vi "Setup_time_windows.vi"() -> ()   [LabVIEW 2017]
uses:
  <vilib>/Utility/file.llb/Read Delimited Spreadsheet (I64).vi
panel:
  in  "x":dbl=25000.0 format="%#_13g"
  out "x/y":dbl=0.25
  out "cal 2":dbl[][](graph)
  out "x-y":dbl
  in  "fine":u64=192 format="%x"
  out "time":dbl=25000.0 format="%.000f"
  in  "通道数量":i32=128
  in  "ch list":u16[](array[numeric])=[0, 1, 6, 7]
  in  "codeDensity":path=path "G:/tdc/2017/test_20240419_071836_codeDensity.csv"
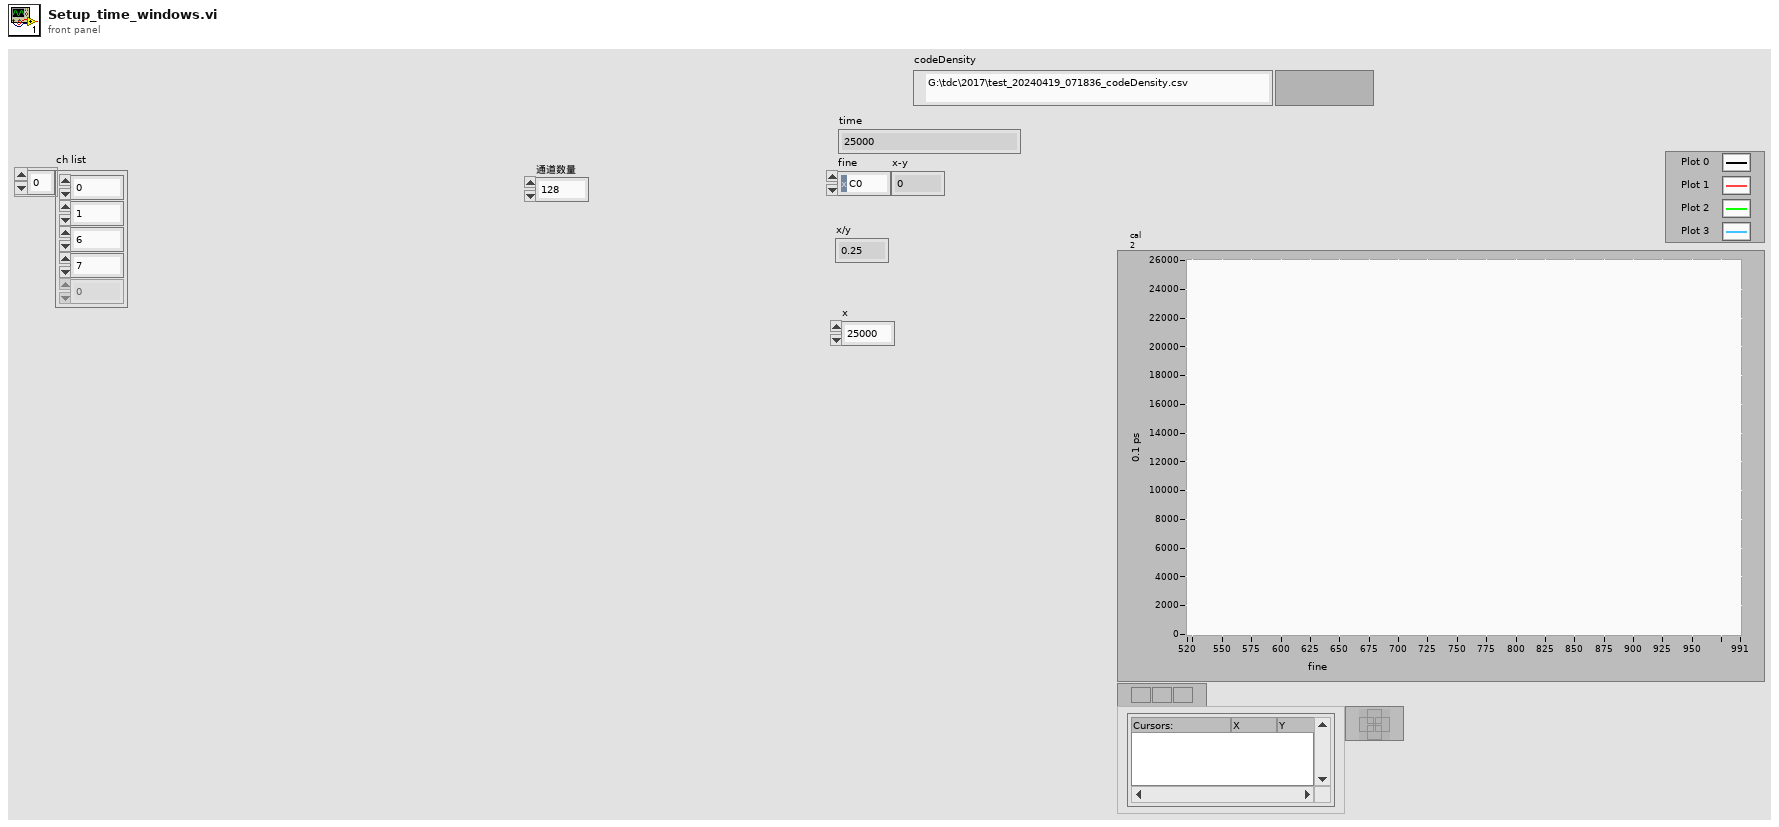
[diagram p1: front panel]
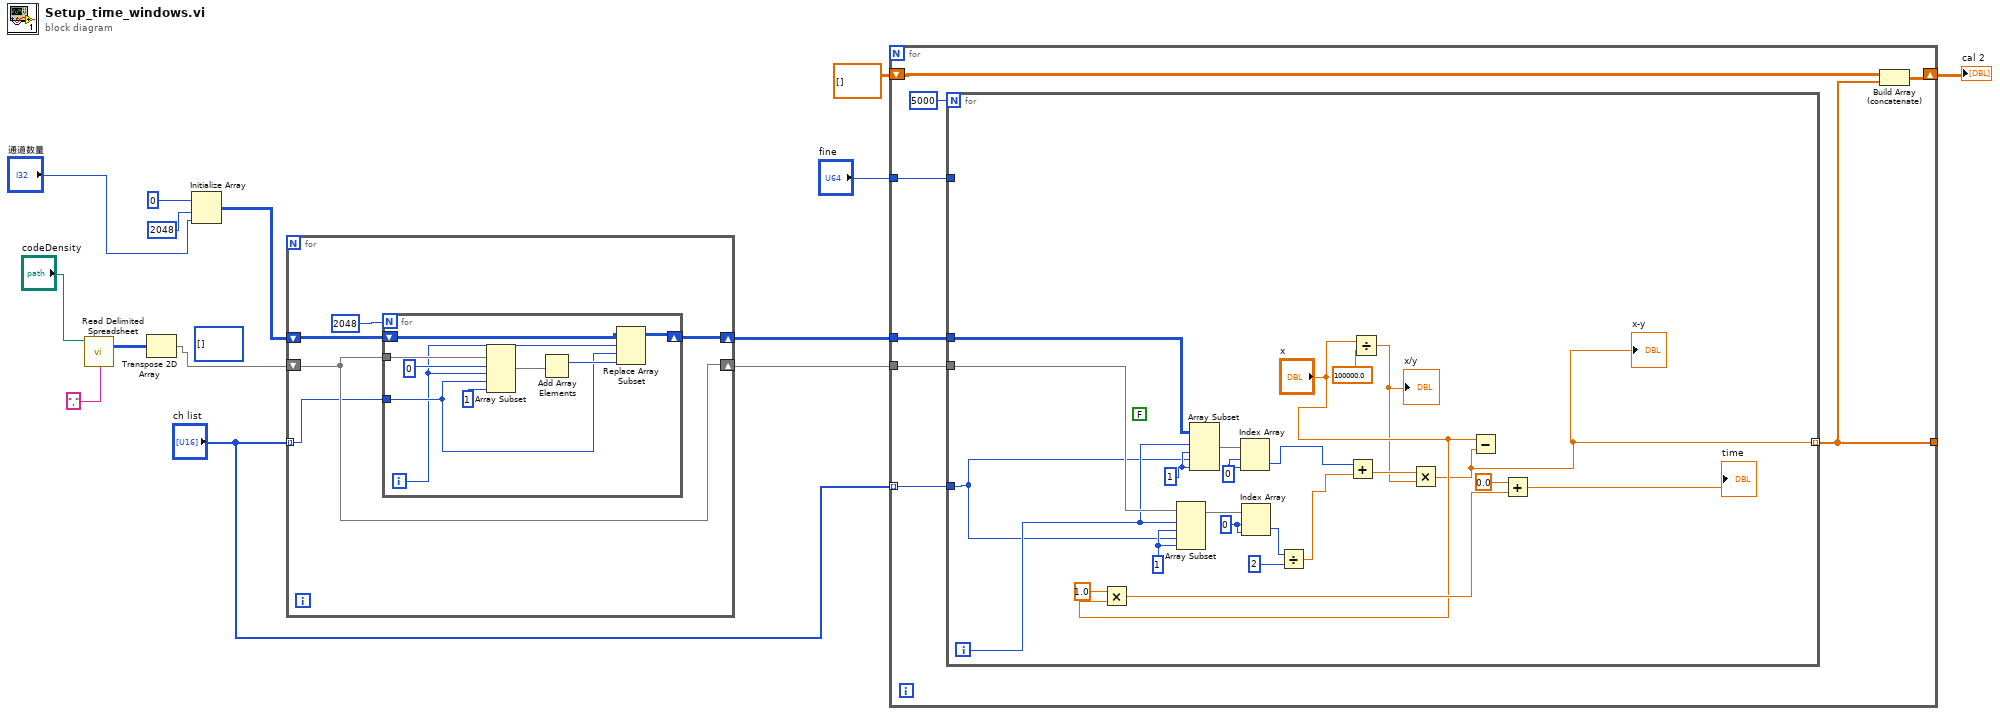
[diagram p0: block diagram]
diagram:
  (unwired) i64[][] []
  n1 = call-poly <vilib>:"Read Delimited Spreadsheet.vi"("file path (dialog if empty)"="codeDensity", "delimiter (\\t)"="," ("delimiter (\\t)")) -> ("all rows"=w14:i64[][])  [unwired: 8 in, 5 out]
  n2 = Transpose 2D Array(2D array=w14) -> (transposed array=w7:i64[][])
  n3 = Initialize Array(u32 0 ("element"), 2048 ("dimension size"), "通道数量") -> (w8:u32[][])
  n4 = for {
    shift-right: [w17] -> w6
    shift-left: w8 -> [w18]
    shift-right: [w16] -> w5
    shift-left: w7 -> [w16]
    tunnel: "ch list" -> [w15] mode=indexing
    n5 = for {
      N: 2048 -> [_]
      tunnel: w16 -> [w28]
      tunnel: w15 -> [w21]
      shift-right: [w23] -> w17
      shift-left: w18 -> [w24]
      i -> [w20]
      n6 = Array Subset(array=w28, index (row)=0 ("索引"), length (row)=w20, index (col)=w21, length (col)=1 ("长度")) -> (w25:i64[][])
      n7 = Add Array Elements(numeric array=w25) -> (sum=w22:i64)
      n8 = Replace Array Subset(array=w24, new element=w22, index (row)=w20, index (col)=w21) -> (w23:u32[][])
    }
  }
  n9 = for {
    tunnel: w6 -> [w36]
    tunnel: w5 -> [w35]
    tunnel: "fine" -> [w34]
    tunnel: [w30] -> _
    tunnel: "ch list" -> [w32] mode=indexing
    shift-right: [w31] -> w1
    shift-left: dbl[][] [] -> [w29]
    n10 = for {
      N: 5000 -> [_]
      tunnel: w36 -> [w42]
      tunnel: w35 -> [w41]
      tunnel: w34 -> [_]
      tunnel: [w38] -> w30 mode=indexing
      tunnel: w32 -> [w37]
      i -> [w39]
      w44 = 0 ("index (row)")
      w46 = 1 ("长度")
      (unwired) FALSE
      w51 = 0 ("索引 (行)")
      w53 = 1 ("长度")
      n11 = Multiply(x=1.0, y="x") -> (x*y=w55:dbl)
      n12 = Array Subset(array=w41, index (row)=w39, length (row)=w53, index (col)=w37, length (col)=w53) -> (w52:i64[][])
      n13 = Array Subset(array=w42, index (row)=w39, length (row)=w46, index (col)=w37, length (col)=w46) -> (w45:u32[][])
      n14 = Index Array(array=w45, index (row)=w44, index (col)=w44) -> (element=w57:u32)
      n15 = Index Array(array=w52, index (row)=w51, index (col)=w51) -> (element=w50:i64)
      n16 = Divide(x=w50, y=u32 2) -> (x/y=w54:dbl)
      n17 = Add(x=w57, y=w54) -> (x+y=w56:dbl)
      n18 = Divide(x="x", y=100000.0) -> (x/y=w48:dbl)
      "x/y" <- w48
      n19 = Multiply(x=w56, y=w48) -> (x*y=w38:dbl)
      "x-y" <- w38
      n20 = Subtract(x="x", y=w38) -> ()  [unwired: 1 out]
      n21 = Add(x=0.0, y=w55) -> (x+y=→"time":dbl)
    }
    n22 = Build Array (concatenate)(w29, w30) -> (w31:dbl[][])
  }
  "cal 2" <- w1
